vi "Open Report File.vi"(8 "error in (no error)":errorcluster, 10 "Path":path, 11 "Mock Report In":refnum<class "Mock Report.lvclass">) -> (0 "error out":errorcluster, 3 "Mock Report Out":refnum<class "Mock Report.lvclass">)   [LabVIEW 2020, in "Mock Report.lvclass"]
uses:
  Mock Report.lvclass
  Mock Report.lvclass/Mock Report.ctl
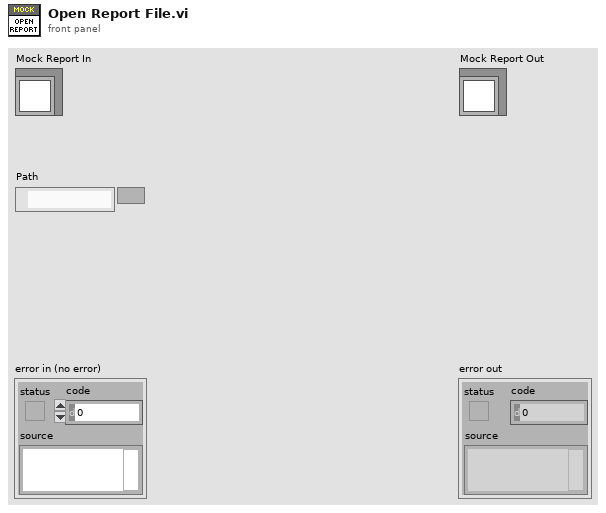
[diagram p1: front panel]
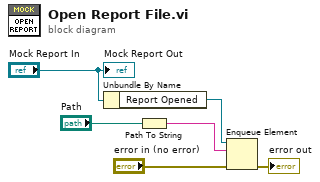
[diagram p0: block diagram]
diagram:
  n1 = Unbundle By Name("Mock Report In") -> ("Report Opened"=w3:refnum<queue>)
  n2 = Path To String(path="Path") -> (string=w1:string)
  n3 = Enqueue Element(queue=w3, element=w1, error in (no error)="error in (no error)") -> (error out=→"error out":errorcluster)  [unwired: 1 in, 2 out]
  "Mock Report Out" <- "Mock Report In"
